vi "FHT.vi"(0 "X":dbl[](array[numeric])) -> (1 "Hartley {X}":dbl[](array[numeric]), 2 "error":i32)   [LabVIEW 2018, in "NI_AALPro.lvlib"]
doc: "Computes the fast Hartley transform (FHT) of the input sequence <B>X</B>."
uses:
  <vilib>/Analysis/NI_AALPro.lvlib
  <resource>/lvanlys.dll
panel:
  # "Fast Hartley Transform"
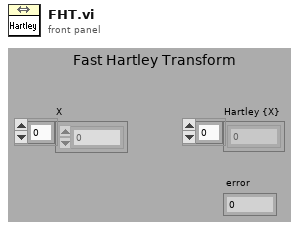
[diagram p1: front panel]
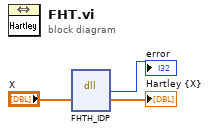
[diagram p0: block diagram]
diagram:
  n1 = dll-call lib="C:/Program Files (x86)/National Instruments/LabVIEW 2018/resource/lvanlys.*" fn="FHTH_IDP"("xH"="X") -> ("return type"=→"error":i32, "xH"=→"Hartley {X}":dbl[])  [unwired: 5 in, 2 out]
